vi "Configure Trigger Level ON Channel.vi"(8 "error in (no error)":errorcluster {"code" format="%.0x"}, 9 "trigger level (0.0 V)":dbl caption="Trigger Level (0.0 V)" format="%^.2e", 10 "Trigger Source (Channel 1)":string(combo)="CHAN1", 11 "VISA Resource Name":refnum<visa-resource-name>) -> (0 "error out":errorcluster {"code" format="%.0x"}, 3 "VISA Resource Name Out":refnum<visa-resource-name>)   [LabVIEW 2011, in "Agilent 546XX Series.lvlib"]
doc: "This VI configures the trigger level for a specified channel.\n\nNOTES:\n\n(1) If a digital channel is selected, the trigger level is set for the entire POD that holds the selected digital channel."
uses:
  Agilent 546XX Series.lvlib
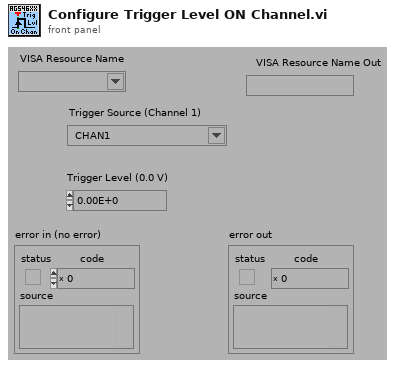
[diagram p1: front panel]
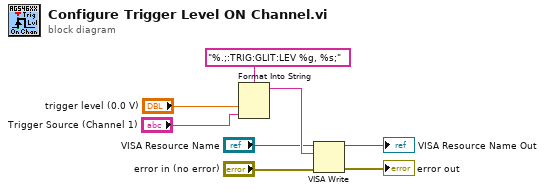
[diagram p0: block diagram]
diagram:
  n1 = Format Into String(format string="%.;:TRIG:GLIT:LEV %g, %s;", "trigger level (0.0 V)", "Trigger Source (Channel 1)") -> (resulting string=w4:string)  [unwired: 2 in, 1 out]
  n2 = VISA Write(VISA resource name="VISA Resource Name", write buffer=w4, error in (no error)="error in (no error)") -> (VISA resource name out=→"VISA Resource Name Out":refnum<visa-resource-name>, error out=→"error out":errorcluster)  [unwired: 1 out]
